vi "SeqMgr.Variables - Get.vi"(8 "error in (no error)":errorcluster, 11 "SeqMgr in":refnum<class "SeqMgr.lvclass">) -> (0 "error out":errorcluster, 2 "Vars":variant, 3 "SeqMgr out":refnum<class "SeqMgr.lvclass">)   [LabVIEW 2024, in "EQMF.lvlib" / "SeqMgr.lvlib" / "SeqMgr.lvclass"]
uses:
  SeqMgr.lvclass
  SeqMgr.lvclass/SeqMgr.ctl
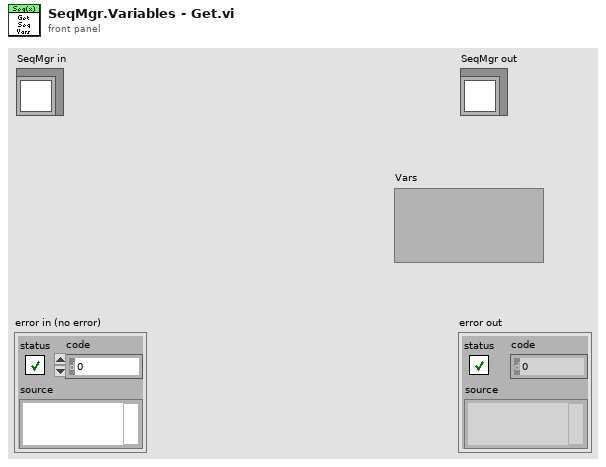
[diagram p1: front panel]
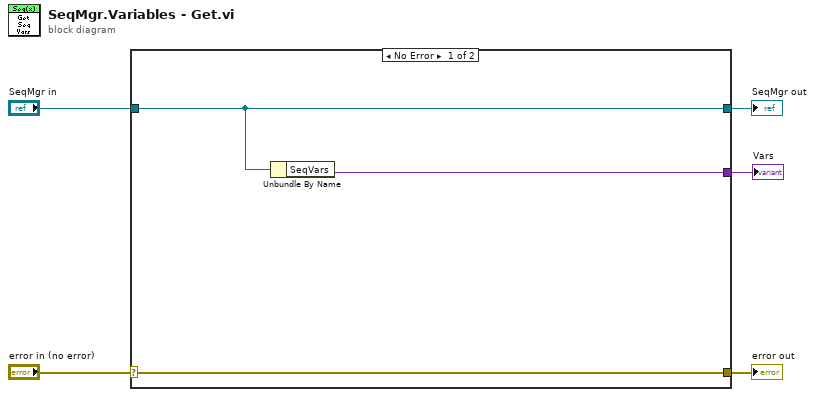
[diagram p0: block diagram]
diagram:
  n1 = case shown="No Error" "error in (no error)" {
    selector: "error in (no error)" -> [w8 w10]
    tunnel: [w8 w10] -> w4
    tunnel: [w6 w9] -> w2
    tunnel: "SeqMgr in" -> [w6 w9]
    tunnel: [w7 _] -> w1
    frame No Error {
      n2 = Unbundle By Name(w6) -> ("SeqVars"=w7:variant)
    }
    frame Error {
    }
  }
  "error out" <- w4
  "SeqMgr out" <- w2
  "Vars" <- w1
